vi "Creators Is Created Event.vi"(10 "Created Event Alias":string, 11 "TEMPLATE Event in":refnum<class "TEMPLATE Event.lvclass">) -> (2 "Is Created Event?":bool, 3 "TEMPLATE Event out":refnum<class "TEMPLATE Event.lvclass">)   [LabVIEW 2021, in "_Template.lvlib" / "Templates.lvlib" / "TEM Event.lvlib" / "TEMPLATE Event.lvclass"]
uses:
  TEMPLATE Event.lvclass
  TEMPLATE Event.lvclass/TEMPLATE Event.ctl
  <vilib>/Nathan Davis/jettl/jettl/Event/Event.lvclass
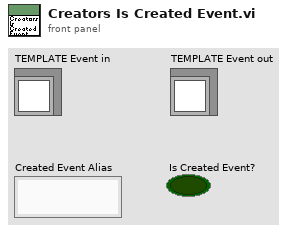
[diagram p1: front panel]
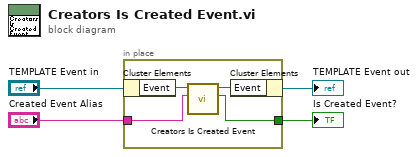
[diagram p0: block diagram]
diagram:
  n1 = in-place {
    in-place-border: [w6] -> w2
    in-place-border: "Created Event Alias" -> [w5]
    n2 = in-place-cluster #1("TEMPLATE Event in") -> ("Event"=w8:refnum<class "Event.lvclass">)
    n3 = call-dynamic "Creators Is Created Event.vi"("Created Event Alias"=w5, "Event in"=w8) -> ("Is Created Event?"=w6:bool, "Event out"=w7:refnum<class "Event.lvclass">)  [unwired: 8 in]
    n4 = in-place-cluster #1("Event"=w7) -> (→"TEMPLATE Event out":refnum<class "TEMPLATE Event.lvclass">)
  }
  "Is Created Event?" <- w2
